vi "Play Sound.vi"(8 "error in (no error)":errorcluster, 9 "Enable Sound":bool, 10 "Volume":dbl(knob) scale=0.0..2000.0, 11 "Electrophysiology in":refnum<class "Electrophysiology.lvclass">) -> (0 "error out":errorcluster, 3 "Electrophysiology out":refnum<class "Electrophysiology.lvclass">)   [LabVIEW 2010, in "Electrophysiology.lvclass"]
uses:
  Electrophysiology.lvclass
  Electrophysiology.lvclass/Electrophysiology.ctl
  <vilib>/sound2/lvsound2.llb/Sound Output Write (DBL).vi
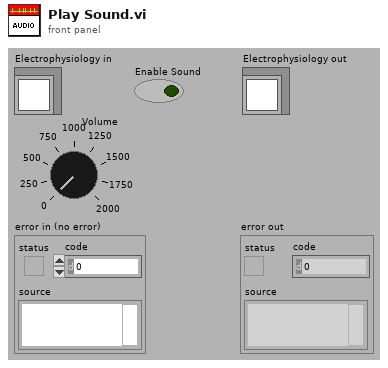
[diagram p1: front panel]
types:
  T1 = typedef "Sound Output Task ID.ctl" = u32
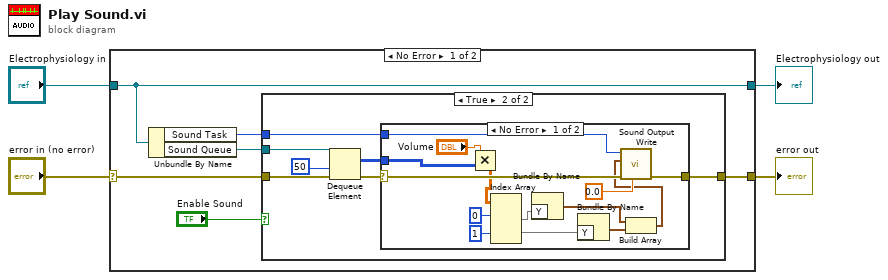
[diagram p0: block diagram]
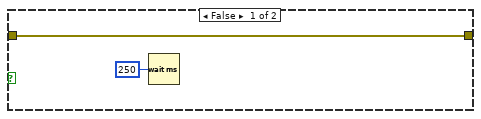
[diagram p2: hidden frame]
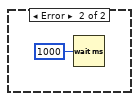
[diagram p3: hidden frame]
diagram:
  n1 = case shown="No Error" "error in (no error)" {
    selector: "error in (no error)" -> [w8 w36]
    tunnel: [w7 w36] -> w3
    tunnel: [w10 w35] -> w1
    tunnel: "Electrophysiology in" -> [w10 w35]
    frame No Error {
      n2 = Unbundle By Name(w10) -> ("Sound Task"=w9:T1, "Sound Queue"=w6:refnum<queue>)
      n3 = case shown="True" "Enable Sound" {
        tunnel: w9 -> [_ w19]
        tunnel: w8 -> [w12 w18]
        tunnel: [w12 w17] -> w7
        tunnel: w6 -> [_ w15]
        frame False {
          n4 = Wait (ms)(milliseconds to wait=u32 250) -> ()  [unwired: 1 out]
        }
        frame True {
          n5 = Dequeue Element(queue=w15, timeout in ms (-1)=u32 50 ("milliseconds to wait"), error in (no error)=w18) -> (element=w16:i32[][], error out=w14:errorcluster)  [unwired: 2 out]
          n6 = case shown="No Error" w14 {
            selector: w14 -> [w28 _]
            tunnel: w19 -> [w32 _]
            tunnel: [w31 _] -> w17
            tunnel: w16 -> [w30 _]
            frame No Error {
              n7 = Multiply(x="Volume", y=w30) -> (x*y=w27:dbl[][])
              n8 = Index Array(array=w27, index (row) #1=0 ("index (row)"), index (row) #2=1 ("index (row)")) -> (element #1=w24:dbl[], element #2=w23:dbl[])  [unwired: 2 in]
              n9 = Bundle By Name("Y"=w24) -> (w21:waveform(dbl))  [unwired: 1 in]
              n10 = Bundle By Name("Y"=w23) -> (w22:waveform(dbl))  [unwired: 1 in]
              n11 = Build Array(w21, w22) -> (w20:waveform(dbl)[])
              n12 = call-poly <vilib>:"Sound Output Write.vi"("timeout (sec)"=0.0, "error in (no error)"=w28, "data"=w20, "task ID"=w32) -> ("error out"=w31:errorcluster)  [unwired: 6 in, 1 out]
            }
            frame Error {
              n13 = Wait (ms)(milliseconds to wait=u32 1000) -> ()  [unwired: 1 out]
            }
          }
        }
      }
    }
    frame Error {
    }
  }
  "error out" <- w3
  "Electrophysiology out" <- w1
